vi "configureConnectorPane.vi"(8 "error in (no error)":errorcluster, 11 "OpenConnectionInstance in":refnum<class "OpenConnectionInstance.lvclass">) -> (0 "error out":errorcluster, 3 "OpenConnectionInstance out":refnum<class "OpenConnectionInstance.lvclass">)   [LabVIEW 2013, in "OpenConnectionInstance.lvclass"]
uses:
  OpenConnectionInstance.lvclass
  PolymorphicInstance/PolymorphicInstance.lvclass/PolymorphicInstance.ctl
  OpenConnectionInstance.lvclass/OpenConnectionInstance.ctl
  PolymorphicInstance/PolymorphicInstance.lvclass
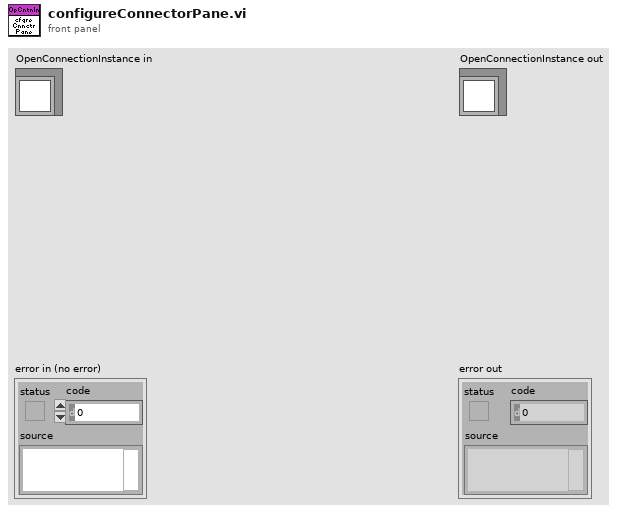
[diagram p1: front panel]
types:
  T1 = enum16{"Invalid Wire Rule", "Required", "Recommended", "Optional", "Dynamic Dispatch"}
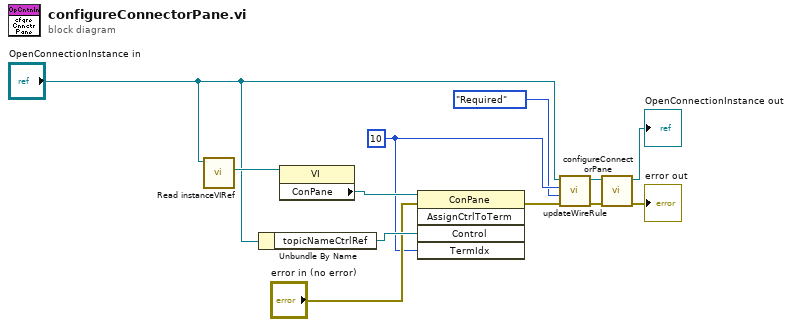
[diagram p0: block diagram]
diagram:
  w6 = u32 10 ("Terminal Index")
  n1 = call "Read instanceVIRef.vi"("PolymorphicInstance in"="OpenConnectionInstance in") -> ("instanceVIRef"=w9:refnum<vi>)  [unwired: 8 in, 2 out]
  n2 = Unbundle By Name("OpenConnectionInstance in") -> ("topicNameCtrlRef"=w8:refnum<vi>)
  n3 = property class="VI"(reference=w9) -> ("ConPane"=w10:refnum<vi>)  [unwired: 1 in, 2 out]
  n4 = invoke class="ConPane" method="AssignCtrlToTerm"(reference=w10, error in="error in (no error)", "Control"=w8, "TermIdx"=w6) -> (error out=w2:errorcluster)  [unwired: 1 in, 4 out]
  n5 = call "updateWireRule.vi"("error in (no error)"=w2, "Wire Rule"=T1."Required", "terminalIndex"=w6, "PolymorphicInstance in"="OpenConnectionInstance in") -> ("error out"=w1:errorcluster, "PolymorphicInstance out"=w3:refnum<class "OpenConnectionInstance.lvclass">)  [unwired: 6 in]
  n6 = call-parent "configureConnectorPane.vi"("error in (no error)"=w1, "PolymorphicInstance in"=w3) -> ("error out"=→"error out":errorcluster, "PolymorphicInstance out"=→"OpenConnectionInstance out":refnum<class "OpenConnectionInstance.lvclass">)  [unwired: 8 in]
